vi "IMG read and QI.vi"() -> ()   [LabVIEW 2017]
panel:
  in  "stop":bool
  out "y_qi 2":sgl
  out "x_qi 2":sgl
  out "rdp_profile":sgl[](array[numeric])
  in  "y_qi":sgl
  in  "x_qi":sgl
  out "Image":T1(plugin-control)
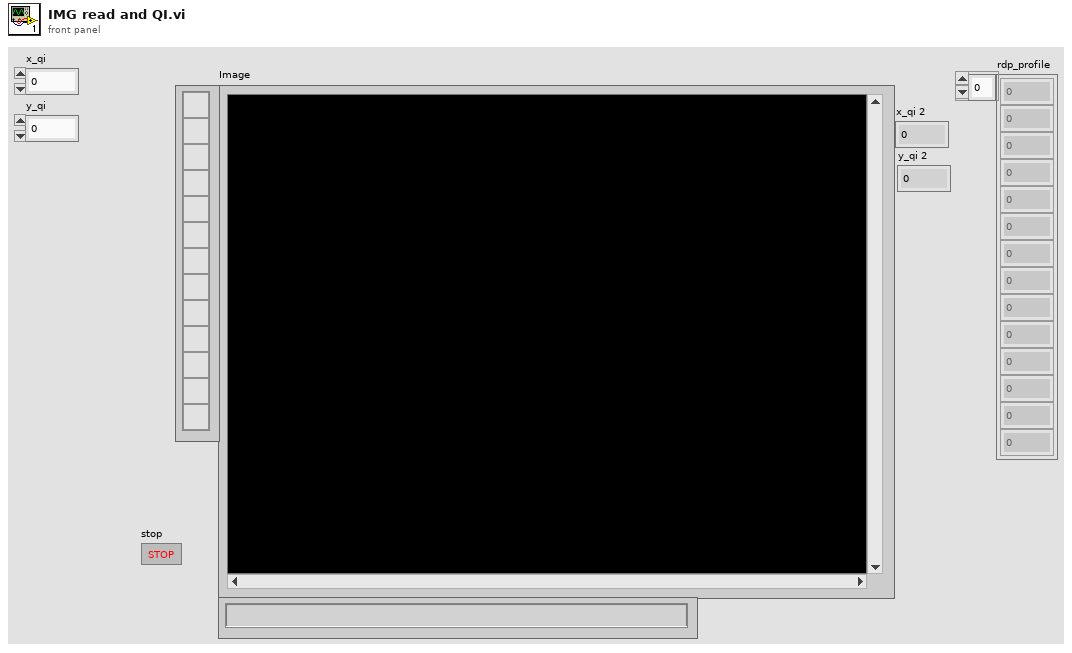
[diagram p1: front panel]
types:
  T1 = typedef "IMAQ Image.ctl" = refnum<image>
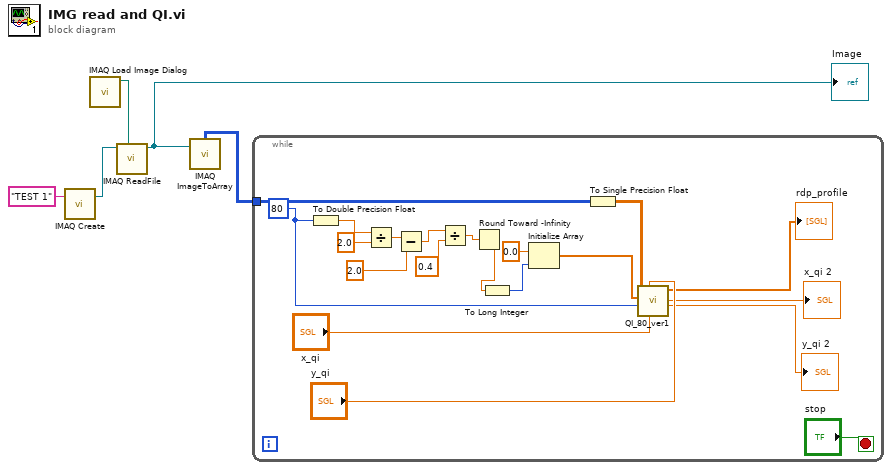
[diagram p0: block diagram]
diagram:
  n1 = call "IMAQ Create"("Image Name"="TEST 1") -> ("New Image"=w4:T1)  [unwired: 4 in, 1 out]
  n2 = call "IMAQ Load Image Dialog"() -> ("Path"=w5:path)  [unwired: 9 in, 2 out]
  n3 = call "IMAQ ReadFile"("File Path"=w5, "Image"=w4) -> ("Image Out"=w2:T1)  [unwired: 5 in, 4 out]
  "Image" <- w2
  n4 = call "IMAQ ImageToArray"("Image"=w2) -> ("Image Pixels (U8)"=w1:u8[][])  [unwired: 3 in, 4 out]
  n5 = while {
    tunnel: w1 -> [w8]
    stop <- "stop" stop-if-true
    w18 = 80 ("arraySize")
    n6 = To Double Precision Float(number=w18) -> (double precision float=w17:dbl)
    n7 = Divide(x=w17, y=2.0) -> (x/y=w15:dbl)
    n8 = Subtract(x=w15, y=2.0) -> (x-y=w13:dbl)
    n9 = Divide(x=w13, y=0.4) -> (x/y=w11:dbl)
    n10 = Round Toward -Infinity(1:w11) -> (0:w10:dbl)
    n11 = To Long Integer(number=w10) -> (32bit integer=w9:i32)
    n12 = Initialize Array(sgl 0.0 ("element"), w9) -> (w24:sgl[])
    n13 = To Single Precision Float(number=w8) -> (single precision float=w7:sgl[][])
    n14 = call "QI_80_ver1.vi"("x_qi in"="x_qi", "y_qi in"="y_qi", "arraySize"=w18, "Array 2"=w24, "Array"=w7) -> ("y_qi out"=→"y_qi 2":sgl, "x_qi out"=→"x_qi 2":sgl, "rdp_profile"=→"rdp_profile":sgl[])  [unwired: 4 in]
  }
